vi "ContinuousTempCollection.vi"() -> ()   [LabVIEW 2016]
uses:
  <vilib>/Utility/file.llb/Write Delimited Spreadsheet (DBL).vi
panel:
  out "Waveform Chart":dbl(graph)
  in  "stop":bool
  in  "file path (dialog if empty)":path
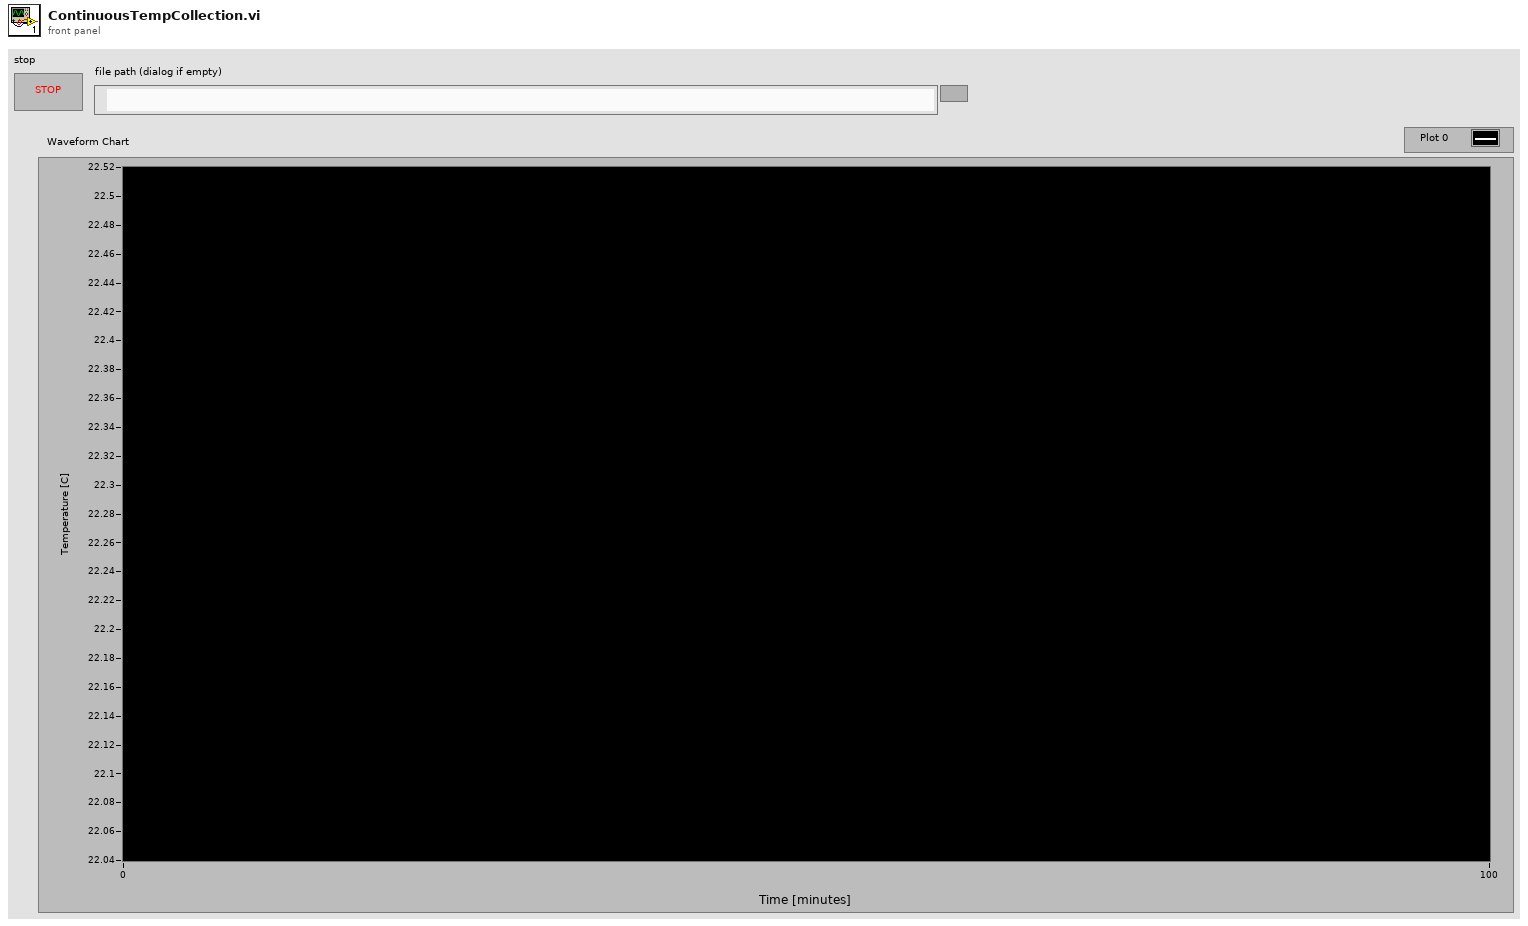
[diagram p1: front panel]
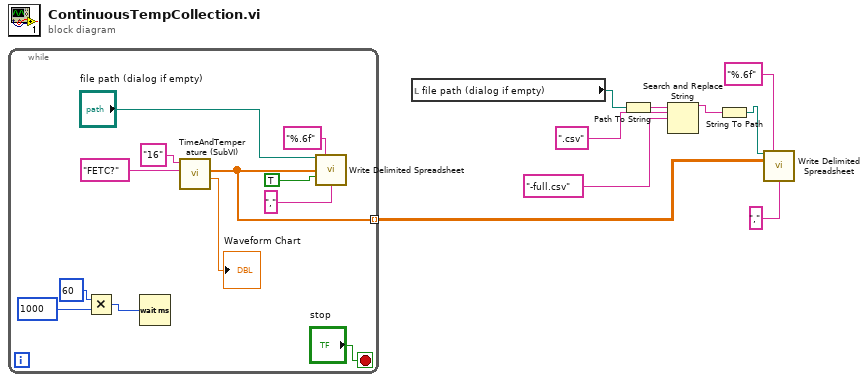
[diagram p0: block diagram]
diagram:
  n1 = while {
    tunnel: [w10] -> w1 mode=indexing
    stop <- "stop" stop-if-true
    n2 = Multiply(x=u32 60 ("milliseconds to wait"), y=u32 1000) -> (x*y=w12:u32)
    n3 = Wait (ms)(milliseconds to wait=w12) -> ()  [unwired: 1 out]
    n4 = call "TimeAndTemperature (SubVI).vi"("Command"="FETC?", "GPIB Address: Temperature"="16") -> ("Temp"=→"Waveform Chart":dbl, "double( Time, Temp )"=w10:dbl[])  [unwired: 6 in, 2 out]
    n5 = call-poly <vilib>:"Write Delimited Spreadsheet.vi"("file path (dialog if empty)"="file path (dialog if empty)", "format (%.3f)"="%.6f", "1D data"=w10, "append to file? (new file:F)"=TRUE, "delimiter (\\t)"="," ("delimiter (\\t)")) -> ()  [unwired: 9 in, 2 out]
  }
  n6 = local read "file path (dialog if empty)"() -> (w9:path)
  n7 = Path To String(path=w9) -> (string=w8:string)
  n8 = Search and Replace String(input string=w8, search string=".csv" ("substring (\"\")"), replace string="-full.csv" ("replace string (\"\")")) -> (result string=w5:string)  [unwired: 5 in, 3 out]
  n9 = String To Path(string=w5) -> (path=w4:path)
  n10 = call-poly <vilib>:"Write Delimited Spreadsheet.vi"("file path (dialog if empty)"=w4, "format (%.3f)"="%.6f", "2D data"=w1, "delimiter (\\t)"="," ("delimiter (\\t)")) -> ()  [unwired: 10 in, 2 out]
